vi "TLPM Find Resources2.vi"(8 "error in (no error)":errorcluster {"code" format="%.0x"}, 11 "instrument handle":refnum<visa-resource-name>) -> (0 "error out":errorcluster {"code" format="%.0x"}, 2 "Resource Count":u32, 3 "instrument handle out":refnum<visa-resource-name>)   [LabVIEW 2023, in "Thorlabs Power Meter.lvlib"]
doc: "This VI finds all driver compatible devices attached to the PC and returns the number of found devices.\n\nNote:\n(1) The VI additionally stores information like system name about the found resources internally. This information can be retrieved with further functions from the class, e.g. <Get Resource Description> and <Get Resource Information>."
uses:
  Thorlabs Power Meter.lvlib
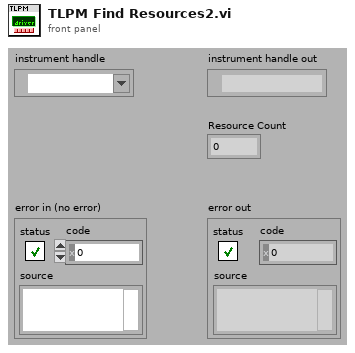
[diagram p1: front panel]
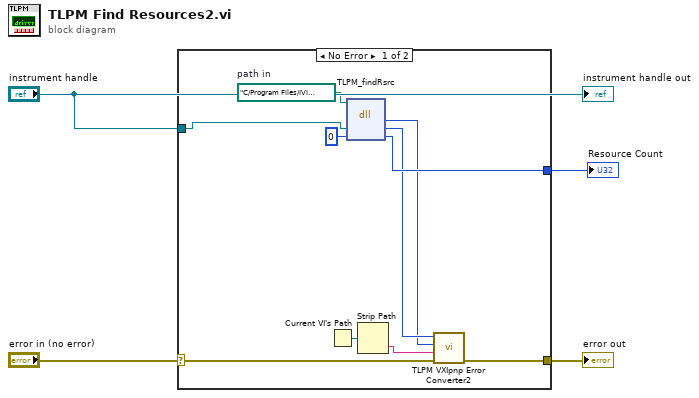
[diagram p0: block diagram]
diagram:
  n1 = case shown="No Error" "error in (no error)" {
    selector: "error in (no error)" -> [w7 w15]
    tunnel: [w6 w15] -> w4
    tunnel: "instrument handle" -> [w13 _]
    tunnel: [w11 _] -> w1
    frame No Error {
      w5 = path "C:/Program Files/IVI Foundation/VISA/Win64/Bin/TLPM_64.dll"  # path in
      n2 = Current VI's Path() -> (path=w14:path)
      n3 = dll-call lib="TLPM_64.dll" fn="TLPM_findRsrc"(path in=w5, "Instrument Handle"=w13, "Resource Count"=u32 0) -> ("return type"=w9:i32, "Instrument Handle"=w10:u32, "Resource Count"=w11:u32)  [unwired: 2 in, 2 out]
      n4 = Strip Path(path=w14) -> (name=w8:string)  [unwired: 1 out]
      n5 = call "TLPM VXIpnp Error Converter2.vi"("error in (no error)"=w7, "Name Of VI (\"\")"=w8, "CVI Error Code (0)"=w9, "instrument handle"=w10) -> ("error out"=w6:errorcluster)  [unwired: 6 in, 1 out]
    }
    frame Error {
    }
  }
  "error out" <- w4
  "Resource Count" <- w1
  "instrument handle out" <- "instrument handle"
